vi "Pulse Mode - Read Setting File Name.vi"(8 "error in (no error)":errorcluster, 11 "VISA resource name":refnum<visa-resource-name>) -> (0 "error out":errorcluster, 2 "File Name":string[](array[string]), 3 "VISA resource name out":refnum<visa-resource-name>)   [LabVIEW 2014, in "Associated Power Technologies 8500 Series.lvlib"]
doc: "Get from instrument the all setting file name on pulse mode."
uses:
  <instrlib>/Associated Power Technologies 8500 Series/Associated Power Technologies 8500 Series.lvlib
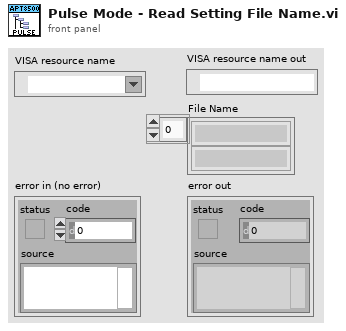
[diagram p1: front panel]
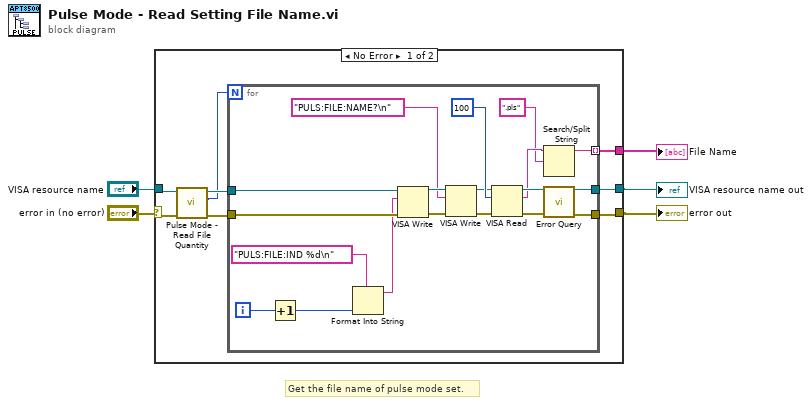
[diagram p0: block diagram]
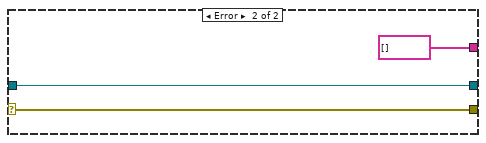
[diagram p2: hidden frame]
diagram:
  # "Get the file name of pulse mode set."
  n1 = case shown="No Error" "error in (no error)" {
    selector: "error in (no error)" -> [w9 w34]
    tunnel: [w12 w34] -> w2
    tunnel: [w13 w35] -> w3
    tunnel: "VISA resource name" -> [w10 w35]
    tunnel: [w11 string[] []] -> w1
    frame No Error {
      n2 = call <instrlib>:"Pulse Mode - Read File Quantity.vi"("error in (no error)"=w9, "VISA resource name"=w10) -> ("error out"=w7:errorcluster, "Total File count"=w6:i32, "VISA resource name out"=w8:refnum<visa-resource-name>)  [unwired: 7 in]
      n3 = for {
        N: w6 -> [_]
        tunnel: w8 -> [w32]
        tunnel: w7 -> [w31]
        tunnel: [w22] -> w13
        tunnel: [w21] -> w12
        tunnel: [w18] -> w11 mode=indexing
        i -> [w15]
        n4 = Increment(x=w15) -> (x+1=w14:i32)
        n5 = Format Into String(format string="PULS:FILE:IND %d\n" ("write buffer"), w14) -> (resulting string=w16:string)  [unwired: 2 in, 1 out]
        n6 = VISA Write(VISA resource name=w32, write buffer=w16, error in (no error)=w31) -> (VISA resource name out=w25:refnum<visa-resource-name>, error out=w24:errorcluster)  [unwired: 1 out]
        n7 = VISA Write(VISA resource name=w25, write buffer="PULS:FILE:NAME?\n", error in (no error)=w24) -> (VISA resource name out=w28:refnum<visa-resource-name>, error out=w29:errorcluster)  [unwired: 1 out]
        n8 = VISA Read(VISA resource name=w28, byte count=u32 100 ("Bytes to Read"), error in (no error)=w29) -> (VISA resource name out=w27:refnum<visa-resource-name>, read buffer=w20:string, error out=w26:errorcluster)  [unwired: 1 out]
        n9 = Search/Split String(string=w20, search string/char (-)=".pls") -> (substring before match=w18:string)  [unwired: 1 in, 2 out]
        n10 = call <instrlib>:"Error Query.vi"("VISA resource name"=w27, "error in (no error)"=w26) -> ("VISA resource name out"=w22:refnum<visa-resource-name>, "error out"=w21:errorcluster)  [unwired: 10 in, 2 out]
      }
    }
    frame Error {
    }
  }
  "VISA resource name out" <- w3
  "error out" <- w2
  "File Name" <- w1
